vi "xPCStopApp.vi"(2 "error in (no error)":errorcluster, 3 "port":i32) -> (0 "error out":errorcluster, 1 "port copy":i32)   [LabVIEW 2018]
uses:
  XPCAPI.DLL
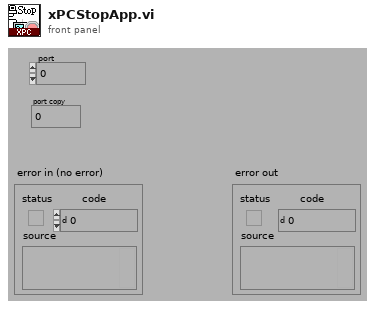
[diagram p1: front panel]
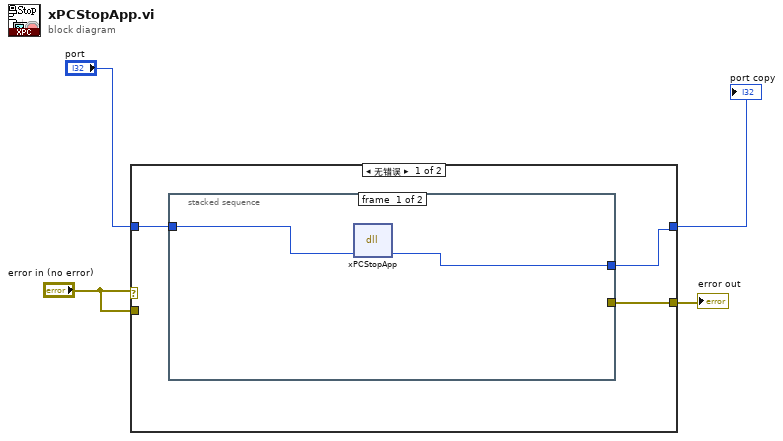
[diagram p0: block diagram]
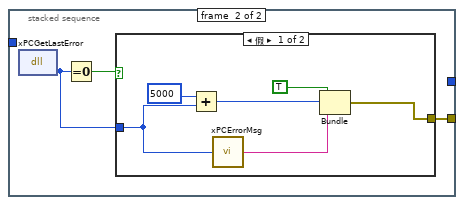
[diagram p2: hidden frame]
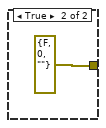
[diagram p3: hidden frame]
diagram:
  n1 = case shown="无错误" "error in (no error)" {
    tunnel: [w7 w21] -> w4
    tunnel: "error in (no error)" -> [_ w21]
    tunnel: "port" -> [w6 w20]
    tunnel: [w5 w20] -> w1
    frame No Error {
      n2 = stacked-sequence {
        tunnel: [w8 _] -> w5
        tunnel: [_ w10] -> w7
        tunnel: w6 -> [w9 _]
        frame #0 {
          n3 = dll-call lib="PTH2Iabs CUsers\nyuchengxinDesktop上下位机联机测试\nxpcapi.dll" fn="xPCStopApp"("port"=w9) -> ("port"=w8:i32)  [unwired: 4 in, 2 out]
        }
        frame #1 {
          n4 = dll-call lib="PTH2Iabs CUsers\nyuchengxinDesktop上下位机联机测试\nxpcapi.dll" fn="xPCGetLastError"() -> (w11:i32)  [unwired: 3 in, 2 out]
          n5 = Equal To 0?(x=w11) -> (x = 0?=w12:bool)
          n6 = case shown="假" w12 {
            tunnel: w11 -> [w14 _]
            tunnel: [w15 errorcluster {"status"=FALSE, "code"=0, "source"=""} ("error out")] -> w10
            frame False {
              n7 = Add(x=5000 ("y"), y=w14) -> (x+y=w17:i32)
              n8 = call "xPCErrorMsg.vi"("error number"=w14) -> ("ErrorMsg"=w16:string)
              n9 = Bundle(TRUE, w17, "ErrorMsg"=w16) -> (w15:cluster{bool, i32, "ErrorMsg":string})  [unwired: 1 in]
            }
            frame True {
            }
          }
        }
      }
    }
    frame Error {
    }
  }
  "port copy" <- w1
  "error out" <- w4
